vi "dfd_Convert QMRate Params to String.vi"(5 "format string":string="%-+024.16e", 6 "width (-)":i16, 7 "indent order":i32, 11 "multirate filter in":T1={"mMRate_Structure"=enum."CIC", "mMRate_Mode"=0, "mMRate_Factor"=1, "mMRate_FIRParams"={"mMRate_FIR_H"=[], "mMRate_FIR_IsNyquist?"=FALSE, "mMRate_FIR_IsSymmetric?"=FALSE}, "mMRate_CICParams"={"mMRate_CIC_#Stage"=2, "mMRate_CIC_Lag"=1, "mMRate_CIC_Type"=enum."Lowpass"}, "mMRate_Order"=1, "mMRate_Version"="1.0", "mMRate_Comments"="1.0", "mMRate_RationalFactor"={"mMRate_L"=-1, "mMRate_M"=-1}, "mMRate_Fs"=0.0, "mMRate_Quantized?"=FALSE, "mMRate_QFilterGain"=1.0, "mMRate_CoefWl"=16, "mMRate_Scaling"={"mMRate_ScaleByPowerOf2?"=FALSE, "mMRate_ScaleType"=enum."Time Domain 1-Norm"}, "mMRate_InputWl"=0, "mMRate_OutputWl"=0, "mMRate_OutputMode"=enum."Nearest", "mMRate_MultMode"=enum."Truncated", "mMRate_BitPruning"=FALSE, "mMRate_GainWl"=16, "mMRate_OutputFwl"=0, "mMRate_SumIwl"=0, "mMRate_InputIwl "=16, "mMRate_SumWl"=32, "mMRate_CoefIwl"=0} {"mMRate_SumWl" min=1 max=32 step=1; "mMRate_InputIwl" min=1 max=32 step=1; "mMRate_GainWl" min=1 max=32 step=1; "mMRate_OutputWl" min=1 max=32 step=1; "mMRate_InputWl" min=1 max=32 step=1; "mMRate_CoefWl" min=1 max=32 step=1; "mMRate_Mode" items=["Default"=-1, "No Rate Change"=0, "Interpolation"=1, "Decimation"=2, "Interpolated"=3, "Rational"=4]}) -> (3 "string":string)   [LabVIEW 2017, in "NI_DigFilter_Process.lvlib"]
uses:
  <vilib>/addons/Digital Filter Design/NI_DigFilter_Process.lvlib
  <vilib>/addons/Digital Filter Design/_Objects.llb/DFD Multirate Filter Obj.ctl
  <vilib>/addons/Digital Filter Design/_Objects.llb/DFD Multirate Mode.ctl
  <vilib>/addons/Digital Filter Design/_Objects.llb/DFD Coef Norm Type.ctl
  <vilib>/addons/Digital Filter Design/_Objects.llb/DFD Round-off Mode.ctl
  <vilib>/addons/Digital Filter Design/_Objects.llb/DFD FXP MRate Multiply Mode.ctl
  <vilib>/addons/Digital Filter Design/NI_DigFilterLicensed.lvlib
  <vilib>/addons/Digital Filter Design/NI_DigFilter_FXP.lvlib
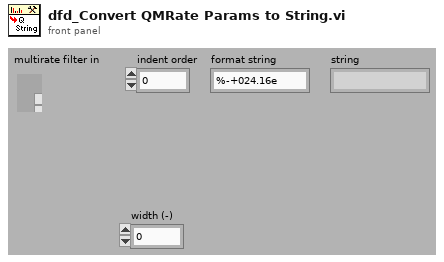
[diagram p1: front panel]
types:
  T1 = typedef "NI_DigFilterLicensed.lvlib/DFD Multirate Filter Obj.ctl" = cluster{"mMRate_Structure":enum16{"CIC", "FIR", "IIR", "Lattice"}, "mMRate_Mode":T2, "mMRate_Factor":i32, "mMRate_FIRParams":cluster{"mMRate_FIR_H":dbl[], "mMRate_FIR_IsNyquist?":bool, "mMRate_FIR_IsSymmetric?":bool}, "mMRate_CICParams":cluster{"mMRate_CIC_#Stage":i32, "mMRate_CIC_Lag":i32, "mMRate_CIC_Type":enum16{"Lowpass", "Highpass"}}, "mMRate_Order":i32, "mMRate_Version":string, "mMRate_Comments":string, "mMRate_RationalFactor":cluster{"mMRate_L":i32, "mMRate_M":i32}, "mMRate_Fs":dbl, "mMRate_Quantized?":bool, "mMRate_QFilterGain":dbl, "mMRate_CoefWl":i16, "mMRate_Scaling":cluster{"mMRate_ScaleByPowerOf2?":bool, "mMRate_ScaleType":T3}, "mMRate_InputWl":i16, "mMRate_OutputWl":i16, "mMRate_OutputMode":T4, "mMRate_MultMode":T5, "mMRate_BitPruning":bool, "mMRate_GainWl":i16, "mMRate_OutputFwl":i16, "mMRate_SumIwl":i16, "mMRate_InputIwl ":i16, "mMRate_SumWl":i16, "mMRate_CoefIwl":i16}
  T2 = typedef "NI_DigFilterLicensed.lvlib/DFD Multirate Mode.ctl" = i16
  T3 = typedef "NI_DigFilterLicensed.lvlib/DFD Coef Norm Type.ctl" = enum16{"No Norm", "Time Domain 1-Norm", "Time Domain 2-Norm", "Time Domain Inf-Norm"}
  T4 = typedef "NI_DigFilterLicensed.lvlib/DFD Round-off Mode.ctl" = enum16{"Nearest", "Truncation"}
  T5 = typedef "NI_DigFilterLicensed.lvlib/DFD FXP MRate Multiply Mode.ctl" = enum16{"Truncated", "Full"}
  T6 = typedef "NI_DigFilterLicensed.lvlib/dfd_Internal Quantization Settings.ctl" = cluster{"source":T7, "wl":i16, "iwl":i16, "overflow mode":enum16{"Saturation", "Wrap"}, "rounding mode":enum16{"Nearest", "Truncation"}, "signed?":bool}
  T7 = typedef "NI_DigFilterLicensed.lvlib/dfd_Internal Quantization Srcs.ctl" = u16
  T8 = typedef "NI_DigFilterLicensed.lvlib/DFD Quantization Settings.ctl" = cluster{"source":T9, "wl":i16, "iwl":i16, "overflow mode":enum16{"Saturation", "Wrap"}, "rounding mode":enum16{"Nearest", "Truncation"}, "signed?":bool}
  T9 = typedef "NI_DigFilterLicensed.lvlib/DFD Quantization Sources.ctl" = u16
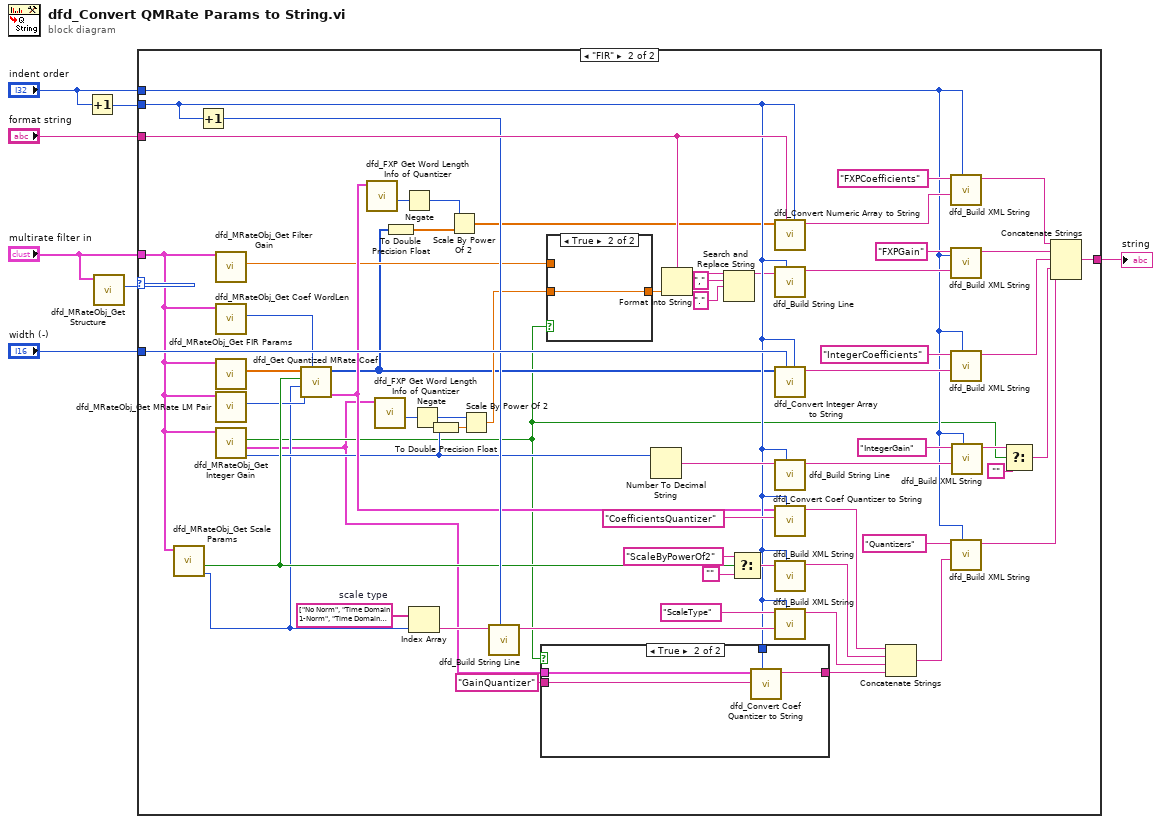
[diagram p0: block diagram]
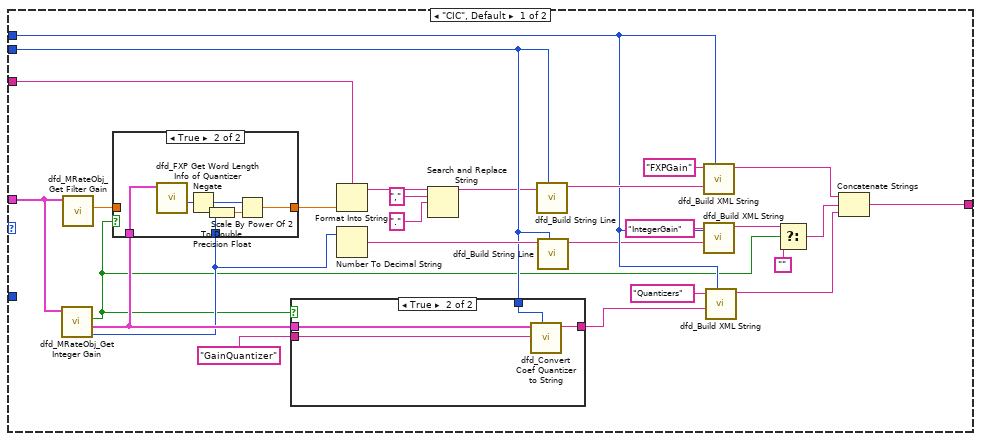
[diagram p2: hidden frame]
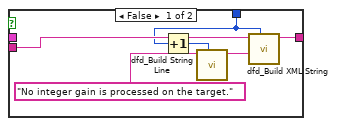
[diagram p3: hidden frame]
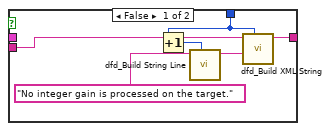
[diagram p5: hidden frame]
diagram:
  n1 = Increment(x="indent order") -> (x+1=w2:i32)
  n2 = call <vilib>:"dfd_MRateObj_Get Structure.vi"("multirate filter in"="multirate filter in") -> ("structure"=w6:enum16{"CIC", "FIR", "IIR", "Lattice"})  [unwired: 10 out]
  n3 = case shown="\"FIR\"" w6 {
    tunnel: "multirate filter in" -> [w30 w78]
    tunnel: "width (-)" -> [_ w112]
    tunnel: "indent order" -> [w28 w85]
    tunnel: [w31 w113] -> w1
    tunnel: w2 -> [w21 w83]
    tunnel: "format string" -> [w34 w105]
    frame "CIC", Default {
      n4 = call <vilib>:"dfd_MRateObj_Get Integer Gain.vi"("multirate filter"=w30) -> ("I32 gain"=w19:i32, "Gain quantizer"=w20:T6, "on FPGA?"=w14:bool)  [unwired: 8 out]
      n5 = call <vilib>:"dfd_MRateObj_Get Filter Gain.vi"("multirate filter in"=w30) -> ("gain"=w23:dbl)  [unwired: 10 out]
      n6 = case shown="True" w14 {
        tunnel: w23 -> [w45 _]
        tunnel: [w45 w47] -> w22
        tunnel: w19 -> [_ w48]
        tunnel: w20 -> [_ w46]
        frame False {
        }
        frame True {
          n7 = call <vilib>:"dfd_FXP Get Word Length Info of Quantizer.vi"("quantization settings"=w46) -> ("fwl"=w49:i16)  [unwired: 10 out]
          n8 = Negate(x=w49) -> (-x=w51:i16)
          n9 = To Double Precision Float(number=w48) -> (double precision float=w50:dbl)
          n10 = Scale By Power Of 2(n=w51, x=w50) -> (x*2^n=w47:dbl)
        }
      }
      n11 = case shown="True" w14 {
        tunnel: [w40 w44] -> w12
        tunnel: w21 -> [w37 w43]
        tunnel: w20 -> [_ w42]
        tunnel: "GainQuantizer" ("element name") -> [w39 w41]
        frame False {
          n12 = Increment(x=w37) -> (x+1=w36:i32)
          n13 = call <vilib>:"dfd_Build String Line.vi"("indent order"=w36, "string"="No integer gain is processed on the target." ("string in")) -> ("string line"=w38:string)  [unwired: 9 out]
          n14 = call <vilib>:"dfd_Build XML String.vi"("indent order"=w37, "string in"=w38, "element name"=w39) -> ("xml string out"=w40:string)  [unwired: 1 in, 7 out]
        }
        frame True {
          n15 = call <vilib>:"dfd_Convert Coef Quantizer to String.vi"("indent order"=w43, "quantizer name"=w41, "quantization settings"=w42) -> ("xml string out"=w44:string)  [unwired: 8 out]
        }
      }
      n16 = Format Into String(format string=w34, w22) -> (resulting string=w9:string)  [unwired: 2 in, 1 out]
      n17 = Number To Decimal String(number=w19) -> (decimal integer string=w25:string)  [unwired: 1 out]
      n18 = Search and Replace String(input string=w9, search string=",", replace string="." ("replace string (\"\")")) -> (result string=w8:string)  [unwired: 2 in, 6 out]
      n19 = call <vilib>:"dfd_Build String Line.vi"("indent order"=w21, "string"=w8) -> ("string line"=w32:string)  [unwired: 9 out]
      n20 = call <vilib>:"dfd_Build String Line.vi"("indent order"=w21, "string"=w25) -> ("string line"=w26:string)  [unwired: 9 out]
      n21 = call <vilib>:"dfd_Build XML String.vi"("indent order"=w28, "string in"=w32, "element name"="FXPGain") -> ("xml string out"=w16:string)  [unwired: 2 in, 6 out]
      n22 = call <vilib>:"dfd_Build XML String.vi"("indent order"=w28, "string in"=w26, "element name"="IntegerGain") -> ("xml string out"=w17:string)  [unwired: 2 in, 6 out]
      n23 = call <vilib>:"dfd_Build XML String.vi"("indent order"=w28, "string in"=w12, "element name"="Quantizers") -> ("xml string out"=w27:string)  [unwired: 2 in, 6 out]
      n24 = Select(t=w17, s=w14, f="") -> (s? t:f=w15:string)
      n25 = Concatenate Strings(w16, w15, w27) -> (w31:string)
    }
    frame "FIR" {
      w52 = string[] ["No Norm", "Time Domain 1-Norm", "Time Domain 2-Norm", "Time Domain Inf-Norm"]  # scale type
      n26 = call <vilib>:"dfd_MRateObj_Get Scale Params.vi"("multirate filter in"=w78) -> ("scale type"=w60:T3, "scale by Power of 2?"=w79:bool)  [unwired: 9 out]
      n27 = Increment(x=w83) -> (x+1=w82:i32)
      n28 = call <vilib>:"dfd_MRateObj_Get Filter Gain.vi"("multirate filter in"=w78) -> ("gain"=w69:dbl)  [unwired: 10 out]
      n29 = call <vilib>:"dfd_MRateObj_Get Coef WordLen.vi"("multirate filter in"=w78) -> ("coef wl"=w77:i16)  [unwired: 10 out]
      n30 = call <vilib>:"dfd_MRateObj_Get FIR Params.vi"("multirate filter in"=w78) -> ("h(n)"=w80:dbl[])  [unwired: 10 out]
      n31 = call <vilib>:"dfd_MRateObj_Get MRate LM Pair.vi"("multirate filter in"=w78) -> ("L"=w71:i32)  [unwired: 1 in, 9 out]
      n32 = call <vilib>:"dfd_MRateObj_Get Integer Gain.vi"("multirate filter"=w78) -> ("I32 gain"=w66:i32, "Gain quantizer"=w53:T6, "on FPGA?"=w58:bool)  [unwired: 8 out]
      n33 = call <vilib>:"dfd_Get Quantized MRate Coef.vi"("coef wl"=w77, "L"=w71, "scale type"=w60, "scale by Power of 2?"=w79, "h"=w80) -> ("coef quantizer"=w70:T8, "h (I32)"=w61:i32[])  [unwired: 5 out]
      n34 = call <vilib>:"dfd_FXP Get Word Length Info of Quantizer.vi"("quantization settings"=w70) -> ("fwl"=w73:i16)  [unwired: 10 out]
      n35 = call <vilib>:"dfd_FXP Get Word Length Info of Quantizer.vi"("quantization settings"=w53) -> ("fwl"=w67:i16)  [unwired: 10 out]
      n36 = To Double Precision Float(number=w61) -> (double precision float=w74:dbl[])
      n37 = Negate(x=w73) -> (-x=w62:i16)
      n38 = Index Array(array=w52, index=w60) -> (element=w101:string)
      n39 = Negate(x=w67) -> (-x=w64:i16)
      n40 = To Double Precision Float(number=w66) -> (double precision float=w65:dbl)
      n41 = Scale By Power Of 2(n=w62, x=w74) -> (x*2^n=w72:dbl[])
      n42 = Scale By Power Of 2(n=w64, x=w65) -> (x*2^n=w63:dbl)
      n43 = call <vilib>:"dfd_Build String Line.vi"("indent order"=w82, "string"=w101) -> ("string line"=w98:string)  [unwired: 9 out]
      n44 = case shown="True" w58 {
        tunnel: [w119 w123] -> w88
        tunnel: w83 -> [w114 w122]
        tunnel: w53 -> [_ w121]
        tunnel: "GainQuantizer" ("element name") -> [w118 w120]
        frame False {
          n45 = Increment(x=w114) -> (x+1=w115:i32)
          n46 = call <vilib>:"dfd_Build String Line.vi"("indent order"=w115, "string"="No integer gain is processed on the target." ("string in")) -> ("string line"=w116:string)  [unwired: 9 out]
          n47 = call <vilib>:"dfd_Build XML String.vi"("indent order"=w114, "string in"=w116, "element name"=w118) -> ("xml string out"=w119:string)  [unwired: 1 in, 7 out]
        }
        frame True {
          n48 = call <vilib>:"dfd_Convert Coef Quantizer to String.vi"("indent order"=w122, "quantizer name"=w120, "quantization settings"=w121) -> ("xml string out"=w123:string)  [unwired: 8 out]
        }
      }
      n49 = case shown="True" w58 {
        tunnel: w69 -> [w124 _]
        tunnel: [w124 w125] -> w68
        tunnel: w63 -> [_ w125]
        frame False {
        }
        frame True {
        }
      }
      n50 = Number To Decimal String(number=w66) -> (decimal integer string=w84:string)  [unwired: 1 out]
      n51 = Format Into String(format string=w105, w68) -> (resulting string=w55:string)  [unwired: 2 in, 1 out]
      n52 = Search and Replace String(input string=w55, search string=",", replace string="." ("replace string (\"\")")) -> (result string=w54:string)  [unwired: 2 in, 6 out]
      n53 = Select(t="ScaleByPowerOf2", s=w79, f="") -> (s? t:f=w99:string)
      n54 = call <vilib>:"dfd_Convert Numeric Array to String.vi"("indent order"=w83, "format string"=w105, "numeric array"=w72) -> ("string"=w106:string)  [unwired: 3 in, 5 out]
      n55 = call <vilib>:"dfd_Build String Line.vi"("indent order"=w83, "string"=w54) -> ("string line"=w104:string)  [unwired: 9 out]
      n56 = call <vilib>:"dfd_Convert Integer Array to String.vi"("indent order"=w83, "width (-)"=w112, "I32 values"=w61) -> ("string"=w110:string)  [unwired: 2 in, 6 out]
      n57 = call <vilib>:"dfd_Build String Line.vi"("indent order"=w83, "string"=w84) -> ("string line"=w87:string)  [unwired: 9 out]
      n58 = call <vilib>:"dfd_Convert Coef Quantizer to String.vi"("indent order"=w83, "quantizer name"="CoefficientsQuantizer" ("element name"), "quantization settings"=w70) -> ("xml string out"=w89:string)  [unwired: 8 out]
      n59 = call <vilib>:"dfd_Build XML String.vi"("indent order"=w83, "element name"=w99) -> ("xml string out"=w95:string)  [unwired: 3 in, 6 out]
      n60 = call <vilib>:"dfd_Build XML String.vi"("indent order"=w83, "string in"=w98, "element name"="ScaleType") -> ("xml string out"=w94:string)  [unwired: 2 in, 6 out]
      n61 = Concatenate Strings(w89, w95, w94, w88) -> (w96:string)
      n62 = call <vilib>:"dfd_Build XML String.vi"("indent order"=w85, "string in"=w106, "element name"="FXPCoefficients") -> ("xml string out"=w108:string)  [unwired: 2 in, 6 out]
      n63 = call <vilib>:"dfd_Build XML String.vi"("indent order"=w85, "string in"=w104, "element name"="FXPGain") -> ("xml string out"=w102:string)  [unwired: 2 in, 6 out]
      n64 = call <vilib>:"dfd_Build XML String.vi"("indent order"=w85, "string in"=w110, "element name"="IntegerCoefficients") -> ("xml string out"=w109:string)  [unwired: 2 in, 6 out]
      n65 = call <vilib>:"dfd_Build XML String.vi"("indent order"=w85, "string in"=w96, "element name"="Quantizers") -> ("xml string out"=w90:string)  [unwired: 2 in, 6 out]
      n66 = call <vilib>:"dfd_Build XML String.vi"("indent order"=w85, "string in"=w87, "element name"="IntegerGain") -> ("xml string out"=w76:string)  [unwired: 2 in, 6 out]
      n67 = Select(t=w76, s=w58, f="") -> (s? t:f=w81:string)
      n68 = Concatenate Strings(w108, w102, w109, w81, w90) -> (w113:string)
    }
  }
  "string" <- w1
